vi "Write Test Info.vi"(8 "error in (no error)":errorcluster, 10 "Test Info":T1={"General"={"Location"="840/176", "Operator"="JLee"}, "Doc"={"Shorthand Test Name"="RVIT1", "MRS Code"="EI020", "P6 Test Activity Name"="JST87NE_RVIT1", "Test Plan"="Added the Version section.", "Wiring Diagram"="HW Configuration"}, "Test Setup"={"Series"="N/A", "Test Code"="N/A", "Test Group"="SNL/NM", "Config Type"="Jung.L"}, "Run"={"Temperature"="Ambient", "Voltage"="Norminal", "Attempt"=1, "Test Run"="3AxxxxxA", "Pre-Test Notes"="TK3AxxxxA", "Source Code"="900", "During Environment"="1", "Enable Dropouts"=FALSE}} {"Run"."Attempt" min=1}, 11 "Special Test configuration in":refnum<class "Special Test configuration.lvclass">) -> (0 "error out":errorcluster, 3 "Special Test configuration out":refnum<class "Special Test configuration.lvclass">)   [LabVIEW 2025, in "Special Test.lvlib" / "Special Test configuration.lvclass"]
uses:
  Special Test configuration.lvclass
  Test Info.ctl
  Special Test configuration.lvclass/Special Test configuration.ctl
panel:
  # "(Select the Shorthand Test Name )"
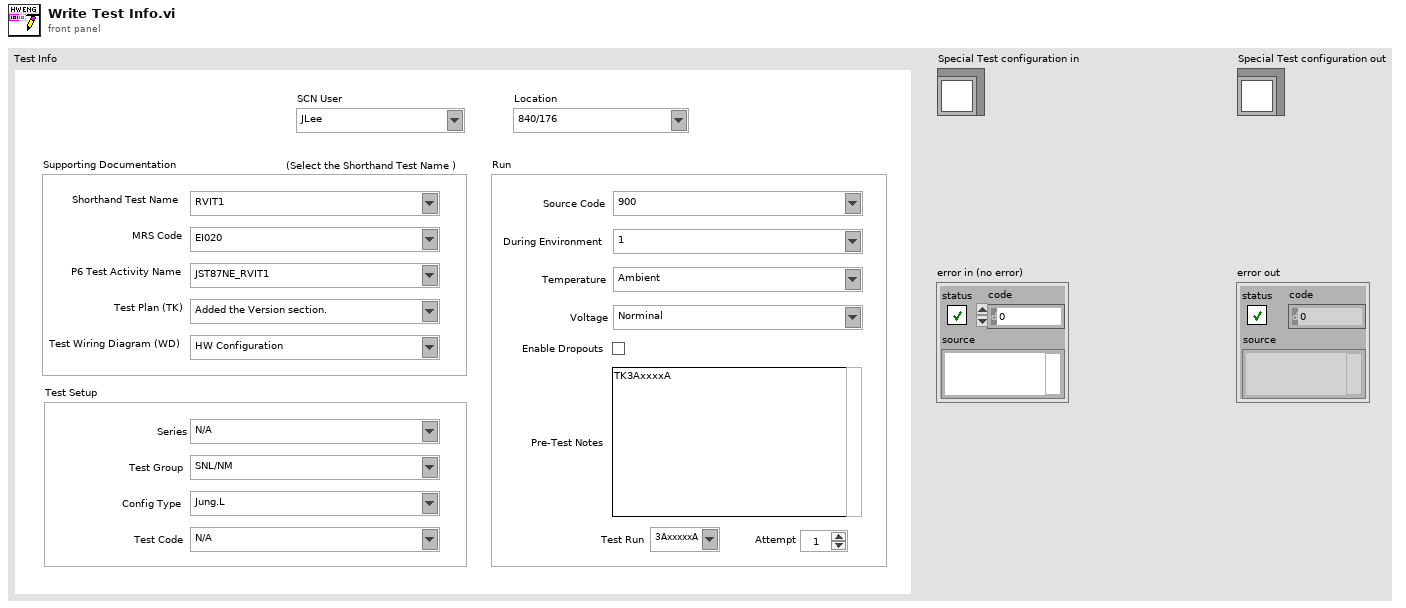
[diagram p1: front panel]
types:
  T1 = typedef "Special Test.lvlib/Special Test configuration.lvclass/Test Info.ctl" = cluster{"General":cluster{"Location":string, "Operator":string}, "Doc":cluster{"Shorthand Test Name":string, "MRS Code":string, "P6 Test Activity Name":string, "Test Plan":string, "Wiring Diagram":string}, "Test Setup":cluster{"Series":string, "Test Code":string, "Test Group":string, "Config Type":string}, "Run":cluster{"Temperature":string, "Voltage":string, "Attempt":u32, "Test Run":string, "Pre-Test Notes":string, "Source Code":string, "During Environment":string, "Enable Dropouts":bool}}
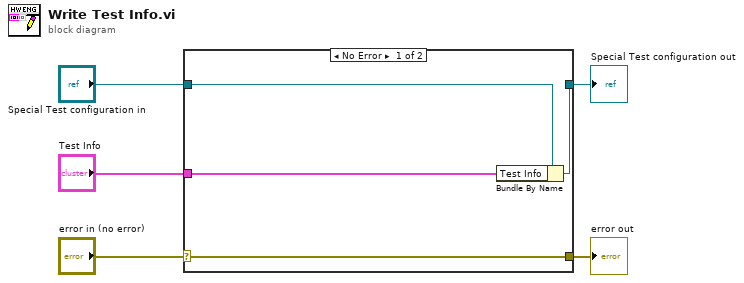
[diagram p0: block diagram]
diagram:
  n1 = case shown="No Error" "error in (no error)" {
    selector: "error in (no error)" -> [w9 w10]
    tunnel: [w9 w10] -> w4
    tunnel: [w7 w11] -> w2
    tunnel: "Special Test configuration in" -> [w8 w11]
    tunnel: "Test Info" -> [w6 _]
    frame No Error {
      n2 = Bundle By Name(cluster=w8, "Test Info"=w6) -> (w7:refnum<class "Special Test configuration.lvclass">)
    }
    frame Error {
    }
  }
  "error out" <- w4
  "Special Test configuration out" <- w2
